vi "BRig_generic_convert__FPGAvalue_to_Voltage__PortAorB_dbl.vi"(11 "input_FPGAvalue_PortAorB":dbl) -> (3 "output_voltage":dbl)   [LabVIEW 2014]
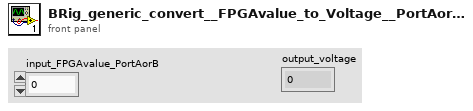
[diagram p1: front panel]
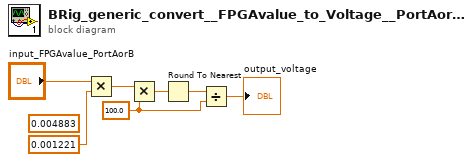
[diagram p0: block diagram]
diagram:
  w4 = 100.0 ("y")
  (unwired) 0.004883 ("f")
  n1 = Multiply(x="input_FPGAvalue_PortAorB", y=0.001221 ("f")) -> (x*y=w7:dbl)
  n2 = Multiply(x=w7, y=w4) -> (x*y=w6:dbl)
  n3 = Round To Nearest(number=w6) -> (nearest integer value=w5:dbl)
  n4 = Divide(x=w5, y=w4) -> (x/y=→"output_voltage":dbl)
